vi "Redis@LPush__Parameter.vi"(1 "ParamterIn":string) -> (0 "ParamterOut":string)   [LabVIEW 2020]
panel:
  in  "Dir=":string(combo)
  in  "Message=":string
  in  "TimeOut=":string(combo)
  in  "Variable=":string(combo)
  in  "Section":string(combo)
  in  "CMD":string
  in  "RedisSession":string(combo)
  in  "Confirm":bool
  # "RedisSession,Value(,Variable=,TimeOut=XXX, Message=XXX,DIr={Start,End})"
  # "@"
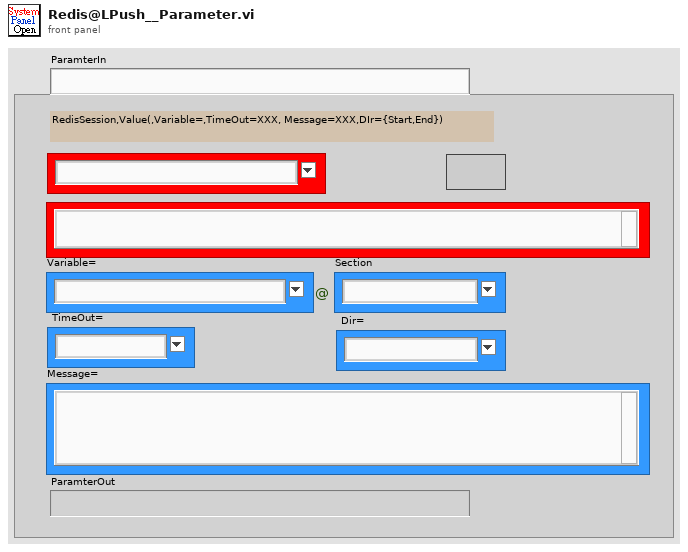
[diagram p1: front panel]
types:
  T1 = enum16{"Get", "Init", "Set", "Delete", "GetElement", "Inc", "Dec"}
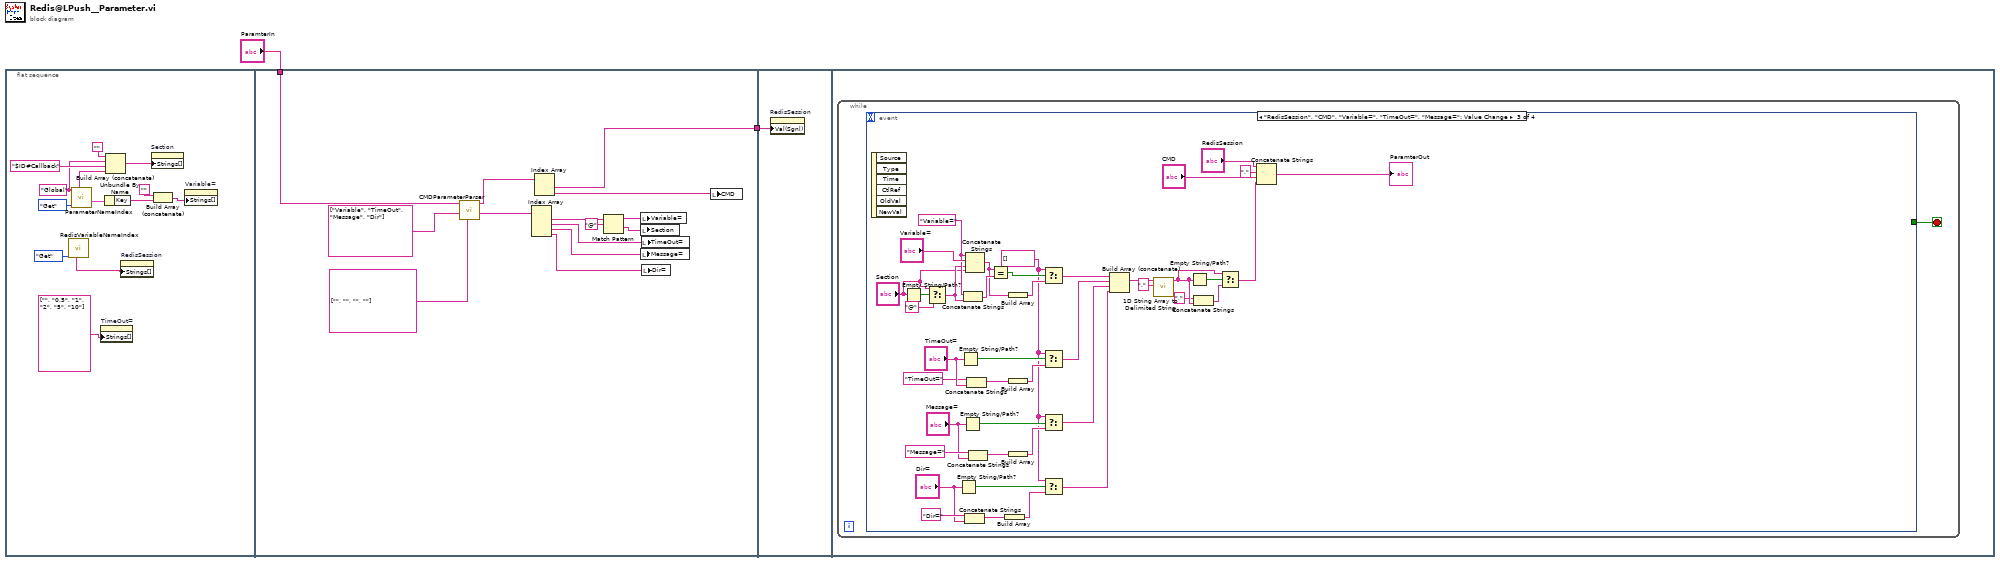
[diagram p0: block diagram]
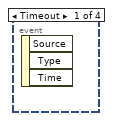
[diagram p2: hidden frame]
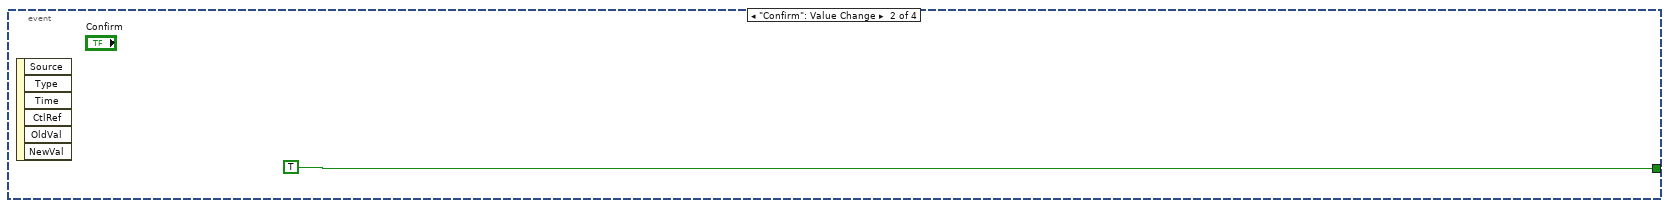
[diagram p3: hidden frame]
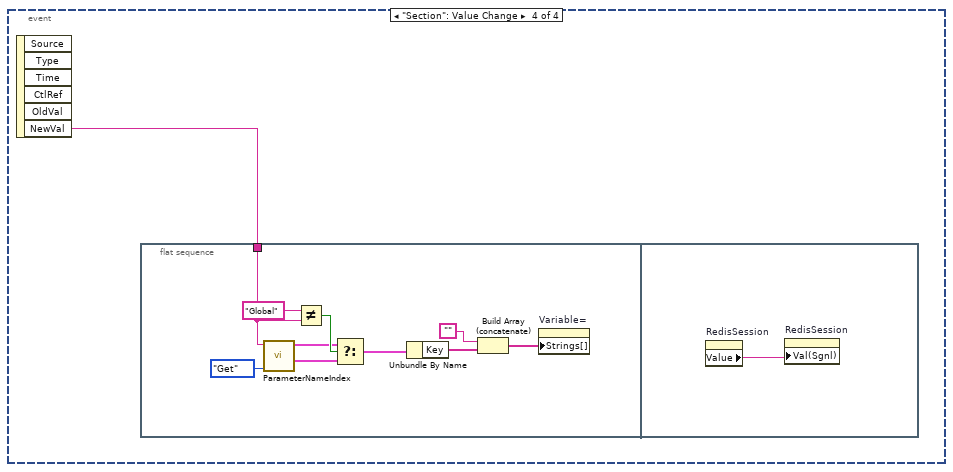
[diagram p4: hidden frame]
diagram:
  n1 = flat-sequence {
    tunnel: "ParamterIn" -> [w29]
    tunnel: [w25] -> w1
    tunnel: w1 -> [w30]
    frame #0 {
      w6 = "Global" ("VariableSection")
      n2 = call "RedisVariableNameIndex.vi"("OP"=enum16{"Add", "Init", "Get"}."Get") -> ("RedisSessionS"=w8:string[])  [unwired: 6 in, 4 out]
      n3 = call "ParameterNameIndex.vi"("OP"=T1."Get", "VariableSection"=w6) -> ("GlobalKeyValue"=w7:cluster{"Key":string[], "Value":string[]}, "SectionList"=w14:string[])  [unwired: 3 in, 5 out]
      n4 = property on="TimeOut=" class="CmbBox"("Strings[]"=string[] ["", "0.5", "1", "2", "5", "10"] ("Strings []")) -> ()  [unwired: 2 in, 2 out]
      n5 = Unbundle By Name(w7) -> ("Key"=w4:string[])
      n6 = Build Array (concatenate)("", w6, "$ID#Callback" ("VariableSection"), w14) -> (w13:string[])
      n7 = property on="RedisSession" class="CmbBox"("Strings[]"=w8) -> ()  [unwired: 2 in, 2 out]
      n8 = property on="Section" class="CmbBox"("Strings[]"=w13) -> ()  [unwired: 2 in, 2 out]
      n9 = Build Array (concatenate)("", w4) -> (w3:string[])
      n10 = property on="Variable=" class="CmbBox"("Strings[]"=w3) -> ()  [unwired: 2 in, 2 out]
    }
    frame #1 {
      n11 = call "CMDParameterParser.vi"("DeafultValues"=string[] ["", "", "", ""], "RequiredKeys"=string[] ["Variable", "TimeOut", "Message", "Dir"], "CMDParameter"=w29) -> ("KeyValues"=w23:string[], "Input"=w26:string[])  [unwired: 6 in, 1 out]
      n12 = Index Array(array=w23) -> (element #1=w22:string, element #2=w19:string, element #3=w18:string, element #4=w16:string)  [unwired: 4 in]
      n13 = Index Array(array=w26) -> (element #1=w25:string, element #2=w24:string)  [unwired: 2 in]
      n14 = Match Pattern(string=w22, regular expression="@") -> (before substring=w20:string, after substring=w17:string)  [unwired: 1 in, 2 out]
      n15 = local write "Variable="(w20) -> ()
      n16 = local write "Section"(w17) -> ()
      n17 = local write "Message="(w18) -> ()
      n18 = local write "TimeOut="(w19) -> ()
      n19 = local write "Dir="(w16) -> ()
      n20 = local write "CMD"(w24) -> ()
    }
    frame #2 {
      n21 = property on="RedisSession" class="CmbBox"("Val(Sgnl)"=w30) -> ()  [unwired: 2 in, 2 out]
    }
    frame #3 {
      n22 = while {
        stop <- w31 stop-if-true
        n23 = event shown="[2] \"RedisSession\", \"CMD\", \"Variable=\", \"TimeOut=\", \"Message=\": Value Change" {
          selector: _ -> [_ _ _ _]
          dyn-events: _ -> [_ _ _ _]
          timeout: _ -> [_ _ _ _]
          tunnel: [_ TRUE _ _] -> w31
          event Timeout {
            n24 = event-data() -> ()  [unwired: 1 in, 3 out]
          }
          event "Confirm": Value Change {
            n25 = event-data() -> ()  [unwired: 1 in, 6 out]
          }
          event "RedisSession", "CMD", "Variable=", "TimeOut=", "Message=": Value Change {
            w34 = string[] [] ("t")
            w67 = "Variable=" ("string")
            n26 = event-data() -> ()  [unwired: 1 in, 6 out]
            n27 = Empty String/Path?(string/path="Section") -> (empty?=w43:bool)
            n28 = Select(t="Section", s=w43, f="@") -> (s? t:f=w41:string)
            n29 = Empty String/Path?(string/path="Dir=") -> (empty?=w36:bool)
            n30 = Empty String/Path?(string/path="TimeOut=") -> (empty?=w66:bool)
            n31 = Empty String/Path?(string/path="Message=") -> (empty?=w61:bool)
            n32 = Concatenate Strings(w67, w41) -> (w60:string)
            n33 = Concatenate Strings("Dir=" ("string"), "Dir=") -> (w39:string)
            n34 = Concatenate Strings(w67, "Variable=", w41, "Section") -> (w44:string)
            n35 = Concatenate Strings("TimeOut=" ("string"), "TimeOut=") -> (w58:string)
            n36 = Concatenate Strings("Message=" ("string"), "Message=") -> (w56:string)
            n37 = Equal?(x=w44, y=w60) -> (x = y?=w68:bool)
            n38 = Build Array(w39) -> (w35:string[])
            n39 = Build Array(w44) -> (w59:string[])
            n40 = Build Array(w58) -> (w57:string[])
            n41 = Build Array(w56) -> (w55:string[])
            n42 = Select(t=w34, s=w68, f=w59) -> (s? t:f=w54:string[])
            n43 = Select(t=w34, s=w66, f=w57) -> (s? t:f=w53:string[])
            n44 = Select(t=w34, s=w61, f=w55) -> (s? t:f=w52:string[])
            n45 = Select(t=w34, s=w36, f=w35) -> (s? t:f=w33:string[])
            n46 = Build Array (concatenate)(w54, w53, w52, w33) -> (w51:string[])
            n47 = call <vilib>:"1D String Array to Delimited String.vi"("delimiter"=",", "string array"=w51) -> ("delimited string"=w48:string)  [unwired: 9 in]
            n48 = Empty String/Path?(string/path=w48) -> (empty?=w49:bool)
            n49 = Concatenate Strings("," ("string"), w48) -> (w46:string)
            n50 = Select(t=w48, s=w49, f=w46) -> (s? t:f=w45:string)
            n51 = Concatenate Strings("RedisSession", "," ("string"), "CMD", w45) -> (→"ParamterOut":string)
          }
          event "Section": Value Change {
            n52 = event-data() -> ("NewVal"=w74:string)  [unwired: 1 in, 5 out]
            n53 = flat-sequence {
              tunnel: w74 -> [w83]
              frame #0 {
                n54 = call "ParameterNameIndex.vi"("OP"=T1."Get", "VariableSection"=w83) -> ("GlobalKeyValue"=w79:cluster{"Key":string[], "Value":string[]}, "SectionKeyValue"=w80:cluster{"Key":string[], "Value":string[]})  [unwired: 3 in, 5 out]
                n55 = Not Equal?(x="Global", y=w83) -> (x != y?=w81:bool)
                n56 = Select(t=w80, s=w81, f=w79) -> (s? t:f=w78:cluster{"Key":string[], "Value":string[]})
                n57 = Unbundle By Name(w78) -> ("Key"=w77:string[])
                n58 = Build Array (concatenate)("", w77) -> (w75:string[])
                n59 = property on="Variable=" class="CmbBox"("Strings[]"=w75) -> ()  [unwired: 2 in, 2 out]
              }
              frame #1 {
                n60 = property on="RedisSession" class="CmbBox"() -> ("Value"=w85:string)  [unwired: 2 in, 2 out]
                n61 = property on="RedisSession" class="CmbBox"("Val(Sgnl)"=w85) -> ()  [unwired: 2 in, 2 out]
              }
            }
          }
        }
      }
    }
  }
